vi "testNumericI64.vi"(8 "error in (no error)":errorcluster, 11 "TestCase in":refnum<class "EasyXMLTest.lvclass">) -> (0 "error out":errorcluster, 3 "TestCase out":refnum<class "EasyXMLTest.lvclass">)   [LabVIEW 2013, in "EasyXMLTest.lvclass"]
doc: "Verify that error in is not overwritten"
uses:
  EasyXMLTest.lvclass
panel:
  out "Generated XML String":string
  out "XML String":string
  out "Input Data":variant
  out "Produced Data":variant
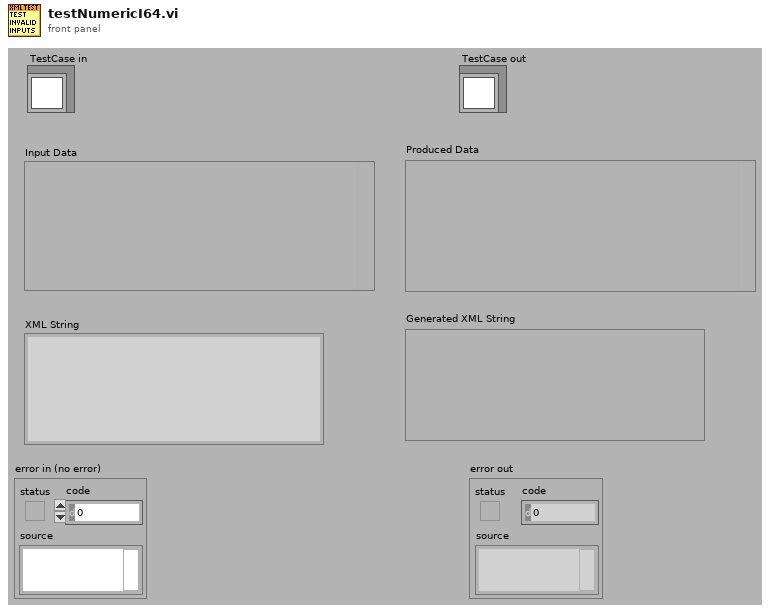
[diagram p1: front panel]
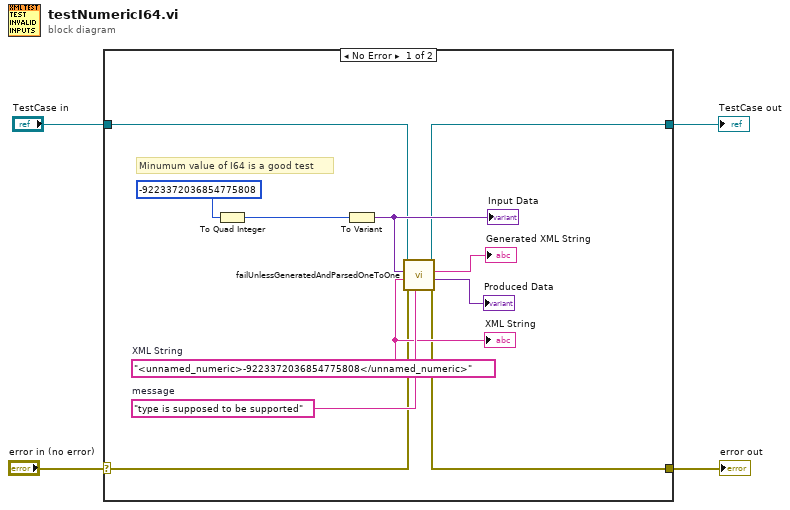
[diagram p0: block diagram]
diagram:
  n1 = case shown="No Error" "error in (no error)" {
    selector: "error in (no error)" -> [w6 w17]
    tunnel: [w7 w17] -> w2
    tunnel: [w8 w16] -> w1
    tunnel: "TestCase in" -> [w5 w16]
    frame No Error {
      w11 = "<unnamed_numeric>-9223372036854775808</unnamed_numeric>"  # XML String
      w15 = "type is supposed to be supported"  # message
      # "Minumum value of I64 is a good test"
      n2 = To Quad Integer(1:i64 -9223372036854775808) -> (0:w9:i64)
      n3 = To Variant(anything=w9) -> (Variant=w13:variant)
      "Input Data" <- w13
      n4 = call "failUnlessGeneratedAndParsedOneToOne.vi"("message (\"\")"=w15, "error in"=w6, "XML String"=w11, "Data"=w13, "EasyXMLTest in"=w5) -> ("error out"=w7:errorcluster, "Produced Data"=→"Produced Data":variant, "Generated XML String"=→"Generated XML String":string, "EasyXMLTest out"=w8:refnum<class "EasyXMLTest.lvclass">)  [unwired: 3 in]
      "XML String" <- w11
    }
    frame Error {
    }
  }
  "error out" <- w2
  "TestCase out" <- w1
